vi "PixieCheckRunStatus.vi"(8 "error in (no error)":errorcluster, 10 "ModNum":u16) -> (0 "error out":errorcluster, 2 "run finished":bool)   [LabVIEW 2013]
uses:
  XIA/Pixie4/Drivers/Pixie4DLL.dll
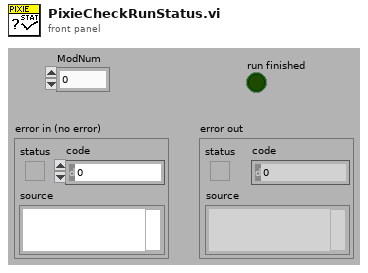
[diagram p1: front panel]
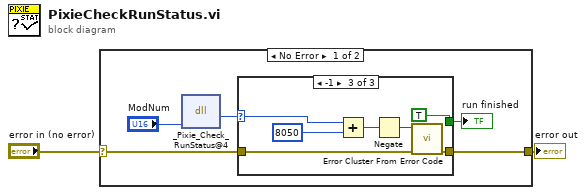
[diagram p0: block diagram]
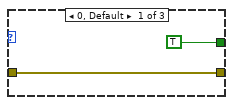
[diagram p2: hidden frame]
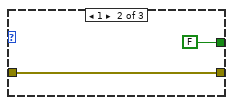
[diagram p3: hidden frame]
diagram:
  n1 = case shown="No Error" "error in (no error)" {
    selector: "error in (no error)" -> [w6 w19]
    tunnel: [w7 w19] -> w1
    frame No Error {
      n2 = dll-call lib="C:/XIA/Pixie4/Drivers/Pixie4DLL.dll" fn="_Pixie_Check_RunStatus@4"("ModNum"="ModNum") -> ("return type"=w4:i32)  [unwired: 4 in, 2 out]
      n3 = case shown="-1" w4 {
        selector: w4 -> [_ _ w13]
        tunnel: [w9 w10 w15] -> w7
        tunnel: w6 -> [w9 w10 w14]
        tunnel: [TRUE ("run active") FALSE ("run active") TRUE ("run active")] -> w3
        frame 0, Default {
        }
        frame 1 {
        }
        frame -1 {
          n4 = Add(x=w13, y=8050) -> (x+y=w17:i32)
          n5 = Negate(x=w17) -> (-x=w16:i32)
          n6 = call <vilib>:"Error Cluster From Error Code.vi"("error in (no error)"=w14, "error code (0)"=w16) -> ("error out"=w15:errorcluster)  [unwired: 1 in, 6 out]
        }
      }
      "run finished" <- w3
    }
    frame Error {
    }
  }
  "error out" <- w1
